vi "Report File Create.vi"(5 "Identifier (\"\")":string, 7 "Append? (T)":bool=TRUE, 8 "error in (no error)":errorcluster, 9 "Open? (T)":bool=TRUE, 10 "Path":path, 11 "Report File in":refnum<class "Report File.lvclass">) -> (0 "error out":errorcluster, 3 "Report File out":refnum<class "Report File.lvclass">)   [LabVIEW 2018, in "Report File.lvclass"]
uses:
  Report File.lvclass
  Report File.lvclass/Report File.ctl
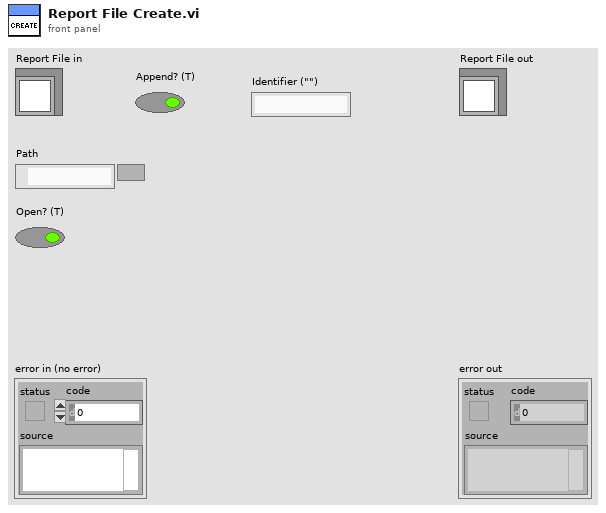
[diagram p1: front panel]
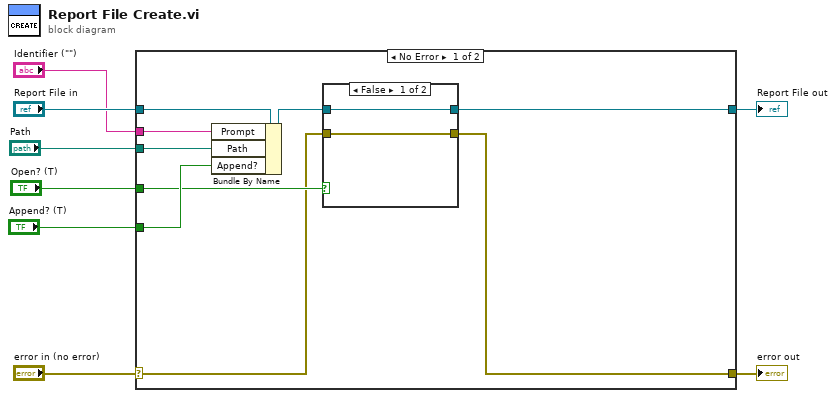
[diagram p0: block diagram]
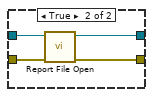
[diagram p2: hidden frame]
diagram:
  n1 = case shown="No Error" "error in (no error)" {
    selector: "error in (no error)" -> [w11 w25]
    tunnel: [w10 w25] -> w7
    tunnel: [w13 w24] -> w5
    tunnel: "Report File in" -> [w17 w24]
    tunnel: "Path" -> [w16 _]
    tunnel: "Open? (T)" -> [w12 _]
    tunnel: "Append? (T)" -> [w15 _]
    tunnel: "Identifier (\"\")" -> [w9 _]
    frame No Error {
      n2 = Bundle By Name(cluster=w17, "Prompt"=w9, "Path"=w16, "Append?"=w15) -> (w14:refnum<class "Report File.lvclass">)
      n3 = case shown="False" w12 {
        tunnel: w14 -> [w18 w23]
        tunnel: [w18 w22] -> w13
        tunnel: w11 -> [w19 w21]
        tunnel: [w19 w20] -> w10
        frame False {
        }
        frame True {
          n4 = call-dynamic "Report File Open.vi"("error in (no error)"=w21, "Report File in"=w23) -> ("error out"=w20:errorcluster, "Report File out"=w22:refnum<class "Report File.lvclass">)  [unwired: 7 in, 1 out]
        }
      }
    }
    frame Error {
    }
  }
  "error out" <- w7
  "Report File out" <- w5
